vi "_PC_MS_SubVI saveData.vi"(6 "ydata":sgl[][](array[numeric]), 7 "File.Save it":refnum<vi>, 8 "error in (no error)":errorcluster, 9 "element":waveform(sgl), 10 "Data Queue":refnum<queue>, 11 "Save_QMH":refnum<class "QMH.lvclass">) -> ()   [LabVIEW 2018]
uses:
  PublicSubVI/Class/QMH/QMH.lvclass
  PublicSubVI/Ctl/RegistyFunc.ctl
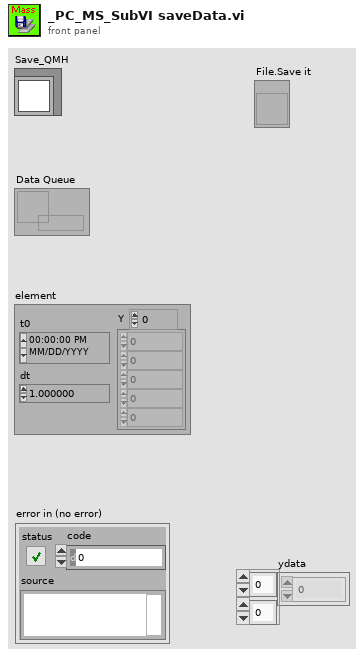
[diagram p1: front panel]
types:
  T1 = enum8{"Enabled", "Disabled", "Disabled and Grayed Out"}
  T2 = enum16{"None", "Init", "Write", "Read", "PauseRead", "FinishCheck"}
  T3 = typedef "RegistyFunc.ctl" = enum16{"None", "FileAutoSave", "FileNoise", "FileSN", "ExeStatu", "WorkFolderPath", "MethodPath", "AVGItem", "LoopItem", "AutoRun", "BGColor", "LineColor", "LineWidth", "XGrid", "YGrid", "DeviceRefnum"}
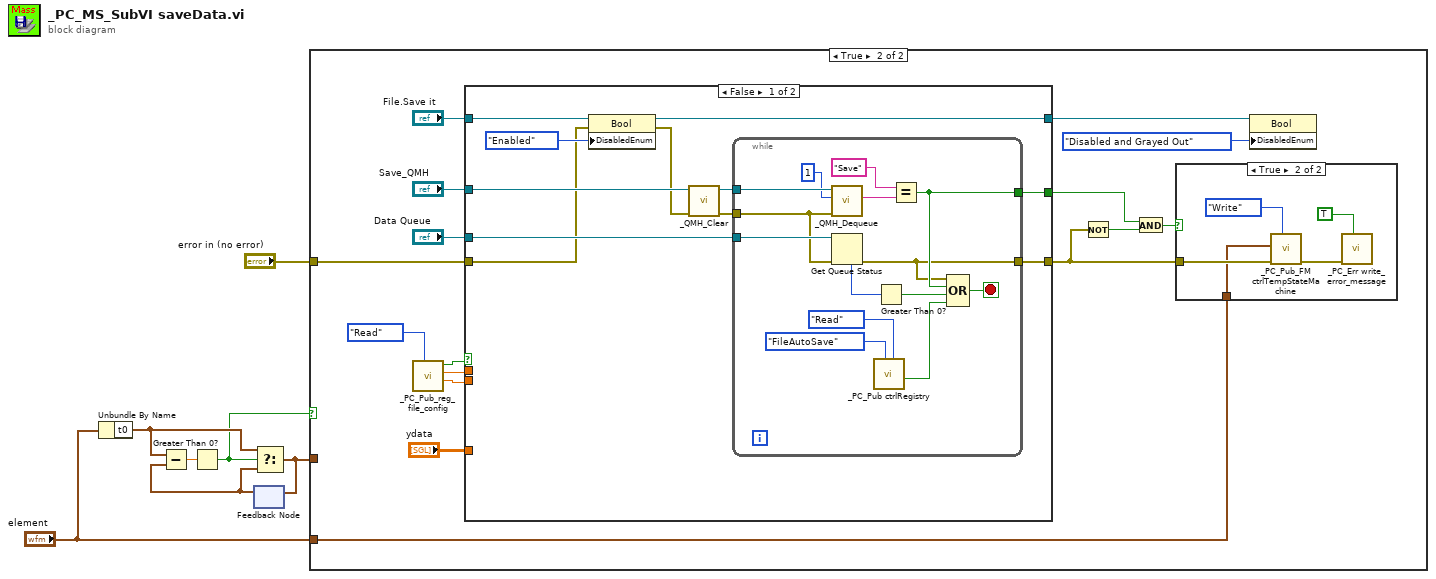
[diagram p0: block diagram]
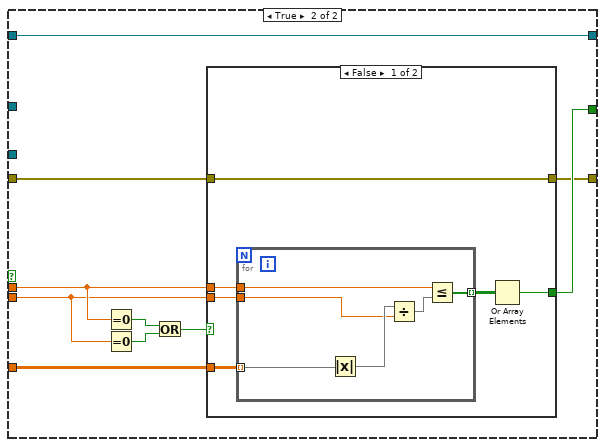
[diagram p4: hidden frame]
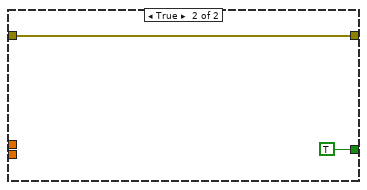
[diagram p5: hidden frame]
diagram:
  n1 = Unbundle By Name("element") -> ("t0"=w5:timestamp)
  n2 = feedback #1() -> (w6:timestamp)  [unwired: 1 in]
  n3 = Subtract(x=w5, y=w6) -> (x-y=w7:dbl)
  n4 = Greater Than 0?(x=w7) -> (x > 0?=w4:bool)
  n5 = Select(t=w5, s=w4, f=w6) -> (s? t:f=w3:timestamp)
  n6 = feedback-in #1(w3) -> ()
  n7 = case shown="True" w4 {
    tunnel: w3 -> [_ _]
    tunnel: "element" -> [_ w8]
    tunnel: "error in (no error)" -> [_ w13]
    frame False {
    }
    frame True {
      n8 = call "_PC_Pub_reg_file_config.vi"("func"=enum16{"None", "Write", "Read"}."Read") -> ("FileSN out"=w15:sgl, "FileNoise out"=w16:dbl, "AutoSave out"=w17:bool)  [unwired: 4 in, 1 out]
      n9 = case shown="False" w17 {
        tunnel: "Save_QMH" -> [w36 _]
        tunnel: [w39 w60] -> w12
        tunnel: "ydata" -> [_ w59]
        tunnel: "Data Queue" -> [w31 _]
        tunnel: "File.Save it" -> [w38 w58]
        tunnel: [w33 w58] -> w19
        tunnel: [w32 w55] -> w9
        tunnel: w16 -> [_ w57]
        tunnel: w15 -> [_ w56]
        tunnel: w13 -> [w29 w54]
        frame False {
          n10 = property class="Bool"(reference=w38, error in=w29, "DisabledEnum"=T1."Enabled" ("Disabled")) -> (reference out=w33:refnum<vi>, error out=w30:errorcluster)
          n11 = call "_QMH_Clear.vi"("error in (no error)"=w30, "QMH in"=w36) -> ("error out"=w34:errorcluster, "QMH out"=w35:refnum<class "QMH.lvclass">)  [unwired: 8 in]
          n12 = while {
            tunnel: w31 -> [w53]
            tunnel: [w45] -> w39
            tunnel: w35 -> [w49]
            tunnel: w34 -> [w44]
            tunnel: [w40] -> w32
            stop <- w51 stop-if-true
            n13 = call "_QMH_Dequeue.vi"("error in (no error)"=w44, "timeout in ms (-1)"=1, "QMH in"=w49) -> ("Msg"=w47:string)  [unwired: 3 in, 5 out]
            n14 = Get Queue Status(queue=w53, error in (no error)=w44) -> (error out=w40:errorcluster, # elements in queue=w52:i32)  [unwired: 1 in, 6 out]
            n15 = call "_PC_Pub ctrlRegistry.vi"("type"=enum16{"None", "Write", "Read"}."Read", "function"=RegistyFunc."FileAutoSave") -> ("Boolean output"=w41:bool)  [unwired: 6 in, 3 out]
            n16 = Greater Than 0?(x=w52) -> (x > 0?=w50:bool)
            n17 = Equal?(x="Save", y=w47) -> (x = y?=w45:bool)
            n18 = Compound Arithmetic op=OR(w40, w45, w50, w41) -> (w51:bool)
          }
        }
        frame True {
          n19 = Equal To 0?(x=w57) -> (x = 0?=w63:bool)
          n20 = Equal To 0?(x=w56) -> (x = 0?=w62:bool)
          n21 = Or(x=w63, y=w62) -> (x .or. y?=w61:bool)
          n22 = case shown="False" w61 {
            tunnel: w57 -> [w69 _]
            tunnel: w56 -> [w68 _]
            tunnel: [w66 TRUE] -> w60
            tunnel: w59 -> [w65 _]
            tunnel: [w64 w76] -> w55
            tunnel: w54 -> [w64 w76]
            frame False {
              n23 = for {
                tunnel: w65 -> [w70] mode=indexing
                tunnel: w68 -> [w73]
                tunnel: w69 -> [w72]
                tunnel: [w71] -> w67 mode=indexing
                n24 = Absolute Value(x=w70) -> (abs(x)=w74:sgl[])
                n25 = Divide(x=w74, y=w73) -> (x/y=w75:sgl[])
                n26 = Less Or Equal?(x=w72, y=w75) -> (x <= y?=w71:bool[])
              }
              n27 = Or Array Elements(Boolean array=w67) -> (logical OR=w66:bool)
            }
            frame True {
            }
          }
        }
      }
      n28 = Not(x=w9) -> (.not. x?=w11:bool)
      n29 = And(x=w12, y=w11) -> (x .and. y?=w10:bool)
      n30 = case shown="True" w10 {
        tunnel: w9 -> [_ w28]
        tunnel: w8 -> [_ w27]
        frame False {
        }
        frame True {
          n31 = call "_PC_Pub_FM ctrlTempStateMachine.vi"("function"=T2."Write", "error in (no error)"=w28, "sourceData"=w27) -> ("error out"=w25:errorcluster)  [unwired: 6 in, 2 out]
          n32 = call "_PC_Err write_error_message.vi"("show msg( T )"=TRUE, "error in"=w25) -> ()  [unwired: 9 in, 1 out]
        }
      }
      n33 = property class="Bool"(reference=w19, "DisabledEnum"=T1."Disabled and Grayed Out" ("Disabled")) -> ()  [unwired: 1 in, 2 out]
    }
  }
